vi "Open.vi"(8 "error in (no error)":errorcluster, 10 "Update Rate (4Hz-100Hz)":u8=100, 11 "navX - I2C in":refnum<class "navX - I2C.lvclass">) -> (0 "error out":errorcluster, 3 "navX - I2C out":refnum<class "navX - I2C.lvclass">)   [LabVIEW 2015, in "navX Library v3.lvlib" / "navX - I2C.lvclass"]
uses:
  navX - I2C.lvclass
  navX - I2C.lvclass/navX - I2C.ctl
  navX - Base/navX - Base.lvclass
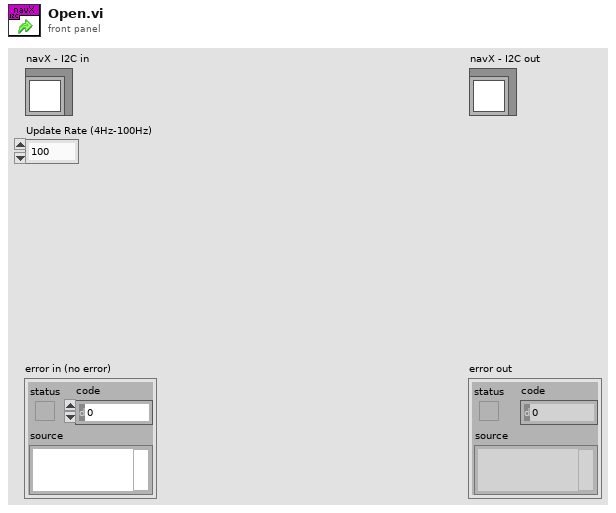
[diagram p1: front panel]
types:
  T1 = typedef "i2c_bus.ctl" = enum16{"I2C On-Board", "I2C MXP", "Invalid"}
  T2 = typedef "WPI_I2CDevRef.ctl" = cluster{"DevStatus":errorcluster, "Device Address":u8, "Handle":i32, "I2C Bus":T1}
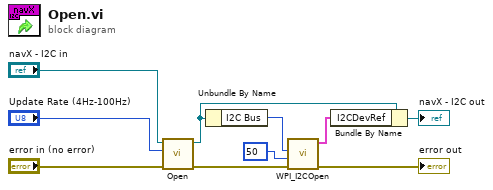
[diagram p0: block diagram]
diagram:
  n1 = call-parent "Open.vi"("error in (no error)"="error in (no error)", "Update Rate (4Hz-100Hz)"="Update Rate (4Hz-100Hz)", "navX - Base in"="navX - I2C in") -> ("error out"=w2:errorcluster, "navX - Base out"=w6:refnum<class "navX - I2C.lvclass">)  [unwired: 7 in]
  n2 = Unbundle By Name(w6) -> ("I2C Bus"=w4:T1)
  n3 = call <vilib>:"WPI_I2COpen.vi"("error in"=w2, "Device Address"=u8 50, "I2C Bus"=w4) -> ("error out"=→"error out":errorcluster, "I2CDevRef"=w3:T2)  [unwired: 7 in]
  n4 = Bundle By Name(cluster=w6, "I2CDevRef"=w3) -> (→"navX - I2C out":refnum<class "navX - I2C.lvclass">)
